vi "GenerateDomains.vi"(6 "Image Dst Out":T2, 7 "Image Type":T1 items=["Grayscale (U8)", "Grayscale (I16)", "Grayscale (SGL)", "Complex (CSG)", "RGB (U32)", "HSL (U32)", "RGB (U64)", "Grayscale (U16)"], 9 "Numeric 2":i32, 10 "Numeric":i32, 11 "Queue in":refnum<queue>) -> (3 "Queue out":refnum<queue>)   [LabVIEW 2019]
uses:
  <vilib>/vision/Image Controls.llb/IMAQ Image.ctl
  <vilib>/vision/NI_Vision_Development_Module.lvlib
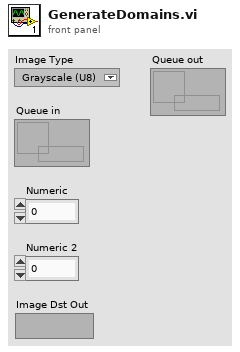
[diagram p1: front panel]
types:
  T1 = typedef "Image Type" = u32
  T2 = typedef "IMAQ Image.ctl" = refnum<image>
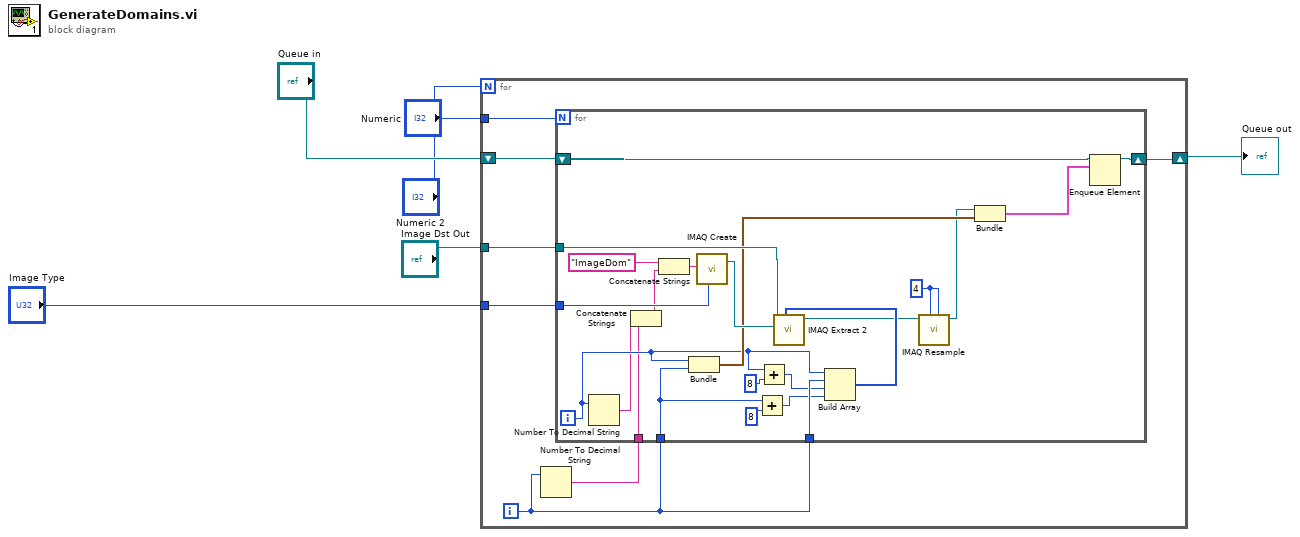
[diagram p0: block diagram]
diagram:
  n1 = for {
    N: "Numeric 2" -> [_]
    tunnel: "Numeric" -> [w13]
    tunnel: "Image Type" -> [w12]
    tunnel: "Image Dst Out" -> [w11]
    shift-right: [w9] -> w6
    shift-left: "Queue in" -> [w10]
    i -> [w8]
    n2 = Number To Decimal String(number=w8) -> (decimal integer string=w7:string)  [unwired: 1 in]
    n3 = for {
      N: w13 -> [_]
      tunnel: w8 -> [w25]
      tunnel: w12 -> [w36]
      tunnel: w11 -> [w34]
      tunnel: w8 -> [w33]
      shift-right: [w21] -> w9
      shift-left: w10 -> [w22]
      tunnel: w7 -> [w18]
      i -> [w20]
      w26 = 4 ("X Resolution")
      n4 = Number To Decimal String(number=w20) -> (decimal integer string=w19:string)  [unwired: 1 in]
      n5 = Concatenate Strings(w19, w18) -> (w17:string)
      n6 = Concatenate Strings("ImageDom" ("Image Name"), w17) -> (w15:string)
      n7 = Bundle(w20, w25) -> (w24:cluster{i32, i32})  [unwired: 1 in]
      n8 = call "IMAQ Create"("Image Name"=w15, "Image Type"=w36) -> ("New Image"=w35:T2)  [unwired: 3 in, 1 out]
      n9 = Add(x=w25, y=8) -> (x+y=w31:i32)
      n10 = Add(x=w20, y=8) -> (x+y=w29:i32)
      n11 = Build Array(w20, w33, w29, w31) -> (w28:i32[])
      n12 = call "IMAQ Extract 2"("Optional Rectangle"=w28, "Image Dst"=w35, "Image Src"=w34) -> ("Image Dst Out"=w27:T2)  [unwired: 7 in, 1 out]
      n13 = call "IMAQ Resample"("X Resolution"=w26, "Y Resolution"=w26, "Image Src"=w27) -> ("Image Dst Out"=w14:T2)  [unwired: 7 in, 1 out]
      n14 = Bundle("Image Dst Out"=w14, w24) -> (w23:cluster{"Image Dst Out":T2, cluster{i32, i32}})  [unwired: 1 in]
      n15 = Enqueue Element(queue=w22, element=w23) -> (queue out=w21:refnum<queue>)  [unwired: 2 in, 2 out]
    }
  }
  "Queue out" <- w6
